vi "Calculate And Insert Biometry Parameter.vi"(8 "error in (no error)":errorcluster caption="错误输入（无错误）", 10 "Measure_No":i64, 11 "connection reference":T1) -> (0 "error out":errorcluster caption="错误输出")   [LabVIEW 2015, in "Boimetry Processing.lvlib"]
doc: "对当初测量第几次的所有测试信号进行计算。\n计算每次生物参数测量结果，测量结果错误判断。计算的结果添加到Biometry的Parameter数据库。\n输入：测量的第几次。"
uses:
  Boimetry Processing.lvlib
  <vilib>/addons/database/Connection.llb/Conn ObjectReference.ctl
  Database Processing/Support/Table/Biometry Parameter.ctl
  Utility VIs/Utility VIs.lvlib
  Digital Signal Processing/Digital Signal Processing.lvlib
  Database Processing/Database Processing.lvlib
  <vilib>/addons/database/NI_Database_API.lvlib
  Digital Image Processing/Digital Image Processing.lvlib
panel:
  # "Busy"
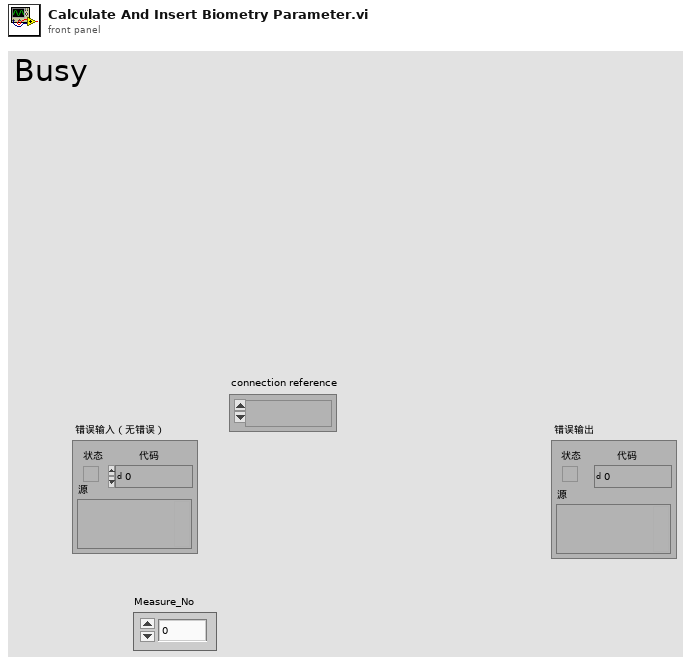
[diagram p1: front panel]
types:
  T1 = typedef "NI_Database_API.lvlib/Conn ObjectReference.ctl" = refnum<k1>
  T2 = typedef "Database Processing.lvlib/Biometry Parameter.ctl" = cluster{"Measure_ID":i64, "Central_Corneal_Thickness":sgl, "Anterior_Chamber_Depth":sgl, "Len_Thickness":sgl, "Retinal_Thickness":sgl, "Axis_Length":sgl, "Pupil_Diameter":sgl, "PCX":sgl, "PCY":sgl, "White_To_White":sgl, "ICX":sgl, "ICY":sgl, "Keratometric_flat":sgl, "Keratometric_steep":sgl, "Keratometric_Axis(flat)":sgl, "Keratometric_Axis(steep)":sgl, "Keratometric_AST":sgl}
  T3 = typedef "Database Processing.lvlib/Biometry Attribute.ctl" = cluster{"Measure_ID":i64, "Measure_No":i64, "Ordinal":i64, "L_Or_R":string}
  T4 = typedef "Digital Signal Processing.lvlib/DSP Configuration.ctl" = cluster{"Sampling Frequency":dbl, "filter type":T5, "RF Filter Low Frequency":dbl, "RF Filter High Frequency":dbl, "RF Filter Taps":i32, "window":T6, "RF window parameter":dbl, "filter type 2":T5, "Demodulated Filter Low Frequency":dbl, "Demodulated Filter HighFrequency":dbl, "Demodulated Filter Order":i32, "SPAN":i32, "Logarithmic Base":dbl, "Noise path":string, "Work position parameter":i32[]}
  T5 = typedef "NI_AALBase.lvlib/Filter Passband Type.ctl" = enum32{"Lowpass", "Highpass", "Bandpass", "Bandstop"}
  T6 = typedef "NI_AALPro.lvlib/windowTd.ctl" = u32
  T7 = typedef "Boimetry Processing.lvlib/Biometry Configuration.ctl" = cluster{"Interference Width":i32, "Interference Threshold":dbl, "Cornea Len Division":i32, "Correction Data 1st Path":string, "1st_Start_Position":dbl, "Correction Data 2nd Path":string, "2nd_Start_Position":dbl, "Index Corneal":dbl, "Index Water":dbl, "Index Len":dbl, "Working Position":cluster{"FirstStart":i32, "FirstEnd":i32, "SecondStart":i32, "SecondEnd":i32}}
  T8 = typedef "Digital Signal Processing.lvlib/DSP Parameter.ctl" = cluster{"RF":cluster{"filter structure":enum32{"IIR 2nd Order", "IIR 4th Order"}, "Reverse Coefficients":dbl[], "Forward Coefficients":dbl[]}, "IIR Filter Cluster":cluster{"filter structure":enum32{"IIR 2nd Order", "IIR 4th Order"}, "Reverse Coefficients":dbl[], "Forward Coefficients":dbl[]}, "Noise Signal":dbl[], "SPAN":i32, "Logarithmic Base":dbl}
  T9 = cluster{"filter structure":enum32{"IIR 2nd Order", "IIR 4th Order"}, "Reverse Coefficients":dbl[], "Forward Coefficients":dbl[]}
  T10 = typedef "Database Processing.lvlib/Biometry Data Path.ctl" = cluster{"Measure_ID":i64, "Ascan_data_Original":string, "picture_pupil_Original":string, "picture_WTW_Original":string, "Ascan_data_Processing":string, "picture_pupil_Processing":string, "picture_WTW_Processing":string, "picture_Processing_K":string, "picture_Processing_ALL":string}
  T11 = cluster{"FirstStart":i32, "FirstEnd":i32, "SecondStart":i32, "SecondEnd":i32}
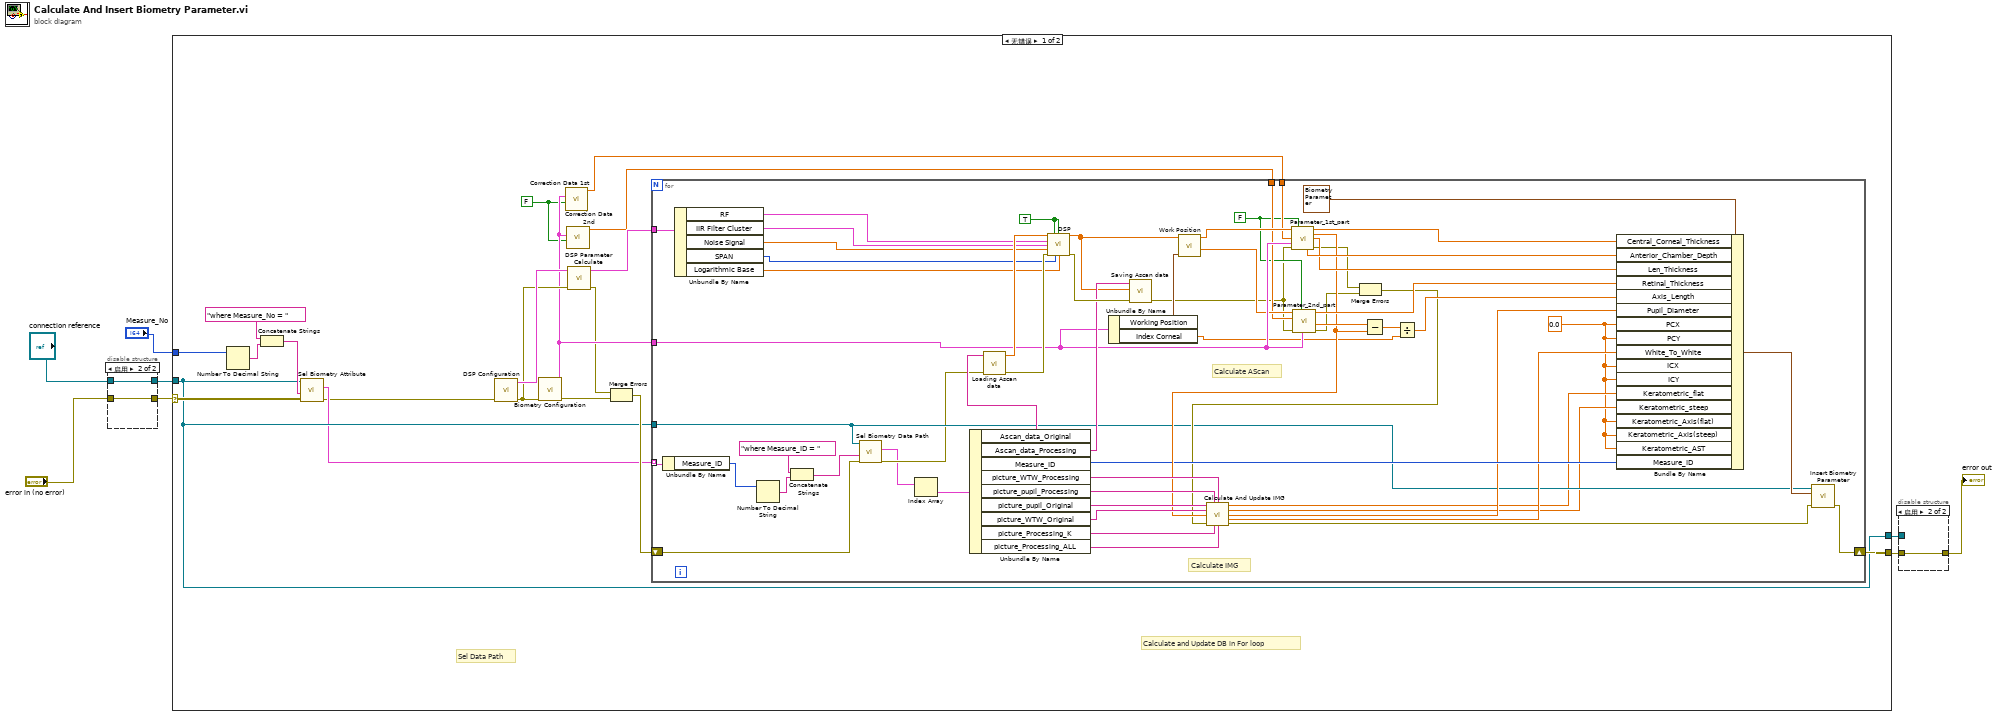
[diagram p0: block diagram]
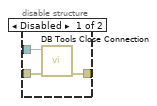
[diagram p2: hidden frame]
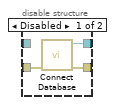
[diagram p3: hidden frame]
diagram:
  n1 = disable-structure shown="启用" {
    disable-tunnel: [w11 w13] -> w8
    disable-tunnel: "error in (no error)" -> [w10 w12]
    disable-tunnel: [w9 w12] -> w6
    disable-tunnel: "connection reference" -> [_ w13]
    frame Disabled {
      n2 = call "Connect Database.vi"("error in (no error)"=w10) -> ("error out"=w9:errorcluster, "connection reference"=w11:T1)  [unwired: 9 in]
    }
    frame Enabled {
    }
  }
  n3 = case shown="无错误" w6 {
    selector: w6 -> [w14 w92]
    tunnel: [w19 w92] -> w4
    tunnel: w8 -> [w16 w91]
    tunnel: [w16 w91] -> w3
    tunnel: "Measure_No" -> [w29 _]
    frame No Error {
      w22 = FALSE ("写入（非为读取）")
      # "Calculate and Update DB in For loop"
      # "Sel Data Path"
      n4 = Number To Decimal String(number=w29) -> (decimal integer string=w31:string)  [unwired: 1 in]
      n5 = Concatenate Strings("where Measure_No = " ("数据库配置.Condition"), w31) -> (w17:string)
      n6 = call "Sel Biometry Attribute.vi"("condition"=w17, "connection reference"=w16) -> ("Biometry Attribute"=w15:T3[])  [unwired: 8 in, 1 out]
      n7 = call "DSP Configuration.vi"("error in (no error)"=w14) -> ("error out"=w26:errorcluster, "DSP Parameter Output"=w28:T4)  [unwired: 9 in]
      n8 = call "Biometry Configuration.vi"("error in (no error)"=w26) -> ("error out"=w20:errorcluster, "Biometry Configuration"=w23:T7)  [unwired: 9 in]
      n9 = call "Correction Data 1st.vi"("写入（非为读取）"=w22, "Biometry Configuration"=w23) -> ("Output Correction Data"=w25:dbl[])  [unwired: 8 in, 1 out]
      n10 = call "Correction Data 2nd.vi"("写入（非为读取）"=w22, "Biometry Configuration"=w23) -> ("Output Correction Data"=w24:dbl[])  [unwired: 8 in, 1 out]
      n11 = call "DSP Parameter Calculate.vi"("error in (no error)"=w26, "DSP Configuration"=w28) -> ("error out"=w21:errorcluster, "DSP Parameter"=w27:T8)  [unwired: 8 in]
      n12 = Merge Errors(w21, w20) -> (w18:errorcluster)
      n13 = for {
        tunnel: w27 -> [w37]
        tunnel: w16 -> [w50]
        tunnel: w23 -> [w74]
        tunnel: w25 -> [w75]
        tunnel: w24 -> [w72]
        shift-right: [w51] -> w19
        shift-left: w18 -> [w49]
        tunnel: w15 -> [w45] mode=indexing
        w38 = sgl 0.0 ("PCX")
        w71 = FALSE
        w90 = TRUE
        # "Calculate IMG"
        # "Calculate AScan"
        n14 = Unbundle By Name(w45) -> ("Measure_ID"=w44:i64)
        n15 = Unbundle By Name(w37) -> ("RF"=w36:T9, "IIR Filter Cluster"=w35:T9, "Noise Signal"=w34:dbl[], "SPAN"=w33:i32, "Logarithmic Base"=w32:dbl)
        n16 = Number To Decimal String(number=w44) -> (decimal integer string=w47:string)  [unwired: 1 in]
        n17 = Concatenate Strings("where Measure_ID = " ("数据库配置.Condition"), w47) -> (w43:string)
        n18 = call "Sel Biometry Data Path.vi"("error in (no error)"=w49, "condition"=w43, "connection reference"=w50) -> ("error out"=w48:errorcluster, "Biometry Data Path"=w42:T10[])  [unwired: 7 in]
        n19 = Index Array(array=w42) -> (element=w41:T10)  [unwired: 1 in]
        n20 = Unbundle By Name(w41) -> ("Ascan_data_Original"=w82:string, "Ascan_data_Processing"=w81:string, "Measure_ID"=w60:i64, "picture_WTW_Processing"=w85:string, "picture_pupil_Processing"=w86:string, "picture_pupil_Original"=w88:string, "picture_WTW_Original"=w87:string, "picture_Processing_K"=w84:string, "picture_Processing_ALL"=w83:string)
        n21 = call "Loading Ascan data.vi"("error in (no error)"=w48, "名称或相对路径"=w82) -> ("error out"=w79:errorcluster, "first row"=w78:dbl[])  [unwired: 8 in]
        n22 = call "DSP.vi"("Input Signal"=w78, "Smooth(F : Don't)"=w90, "Minus Noise(F : Don't)"=w90, "RF"=w36, "IIR Filter Cluster"=w35, "Noise Signal"=w34, "error in (no error)"=w79, "SPAN"=w33, "Logarithmic Base"=w32) -> ("DSP signal"=w77:dbl[], "error out"=w89:errorcluster)  [unwired: 5 in]
        n23 = Unbundle By Name(w74) -> ("Working Position"=w80:T11, "Index Corneal"=w62:dbl)
        n24 = call "Saving Ascan data.vi"("error in (no error)"=w89, "Ascan Data"=w77, "名称或相对路径"=w81) -> ("error out"=w57:errorcluster)  [unwired: 8 in]
        n25 = call "Work Position.vi"("Working Position"=w80, "S"=w77) -> ("S_2nd_part"=w73:dbl[], "S_1st_part"=w76:dbl[])  [unwired: 4 in, 4 out]
        n26 = call "Parameter_1st_part.vi"("S"=w76, "测试"=w71, "Correction Data 1st"=w75, "Biometry Configuration"=w74, "Error In"=w57) -> ("角膜厚度"=w69:dbl, "开始位置"=w64:dbl, "晶体厚度"=w67:dbl, "前方深度"=w68:dbl, "Error Out"=w56:errorcluster)  [unwired: 4 in, 2 out]
        n27 = call "Parameter_2nd_part.vi"("Biometry Configuration"=w74, "测试？"=w71, "Error In"=w57, "Correction Data 2nd"=w72, "S"=w73) -> ("Error Out"=w55:errorcluster, "最值位置"=w65:dbl, "视网膜厚度"=w66:dbl)  [unwired: 3 in, 1 out]
        n28 = Merge Errors(w56, w55) -> (w54:errorcluster)
        n29 = call "Calculate And Update IMG.vi"("pictuer_pupil_Original"=w88, "pictuer_pupil_Processing"=w86, "pictuer_WTW_Processing"=w85, "pictuer_WTW_Original"=w87, "D"=w64, "error in (no error)"=w54, "picture_Processing_K"=w84, "picture_Processing_ALL"=w83) -> ("a"=w40:dbl, "b"=w39:dbl, "PD"=w59:dbl, "WTW"=w58:dbl, "error out"=w52:errorcluster)  [unwired: 3 in]
        n30 = Subtract(x=w65, y=w64) -> (x-y=w63:dbl)
        n31 = Divide(x=w63, y=w62) -> (x/y=w61:dbl)
        n32 = Bundle By Name(cluster=T2 {"Measure_ID"=0, "Central_Corneal_Thickness"=0.0, "Anterior_Chamber_Depth"=0.0, "Len_Thickness"=0.0, "Retinal_Thickness"=0.0, "Axis_Length"=0.0, "Pupil_Diameter"=0.0, "PCX"=0.0, "PCY"=0.0, "White_To_White"=0.0, "ICX"=0.0, "ICY"=0.0, "Keratometric_flat"=0.0, "Keratometric_steep"=0.0, "Keratometric_Axis(flat)"=0.0, "Keratometric_Axis(steep)"=0.0, "Keratometric_AST"=0.0} ("Biometry Parameter"), "Central_Corneal_Thickness"=w69, "Anterior_Chamber_Depth"=w68, "Len_Thickness"=w67, "Retinal_Thickness"=w66, "Axis_Length"=w61, "Pupil_Diameter"=w59, "PCX"=w38, "PCY"=w38, "White_To_White"=w58, "ICX"=w38, "ICY"=w38, "Keratometric_flat"=w40, "Keratometric_steep"=w39, "Keratometric_Axis(flat)"=w38, "Keratometric_Axis(steep)"=w38, "Keratometric_AST"=w38, "Measure_ID"=w60) -> (w53:T2)
        n33 = call "Insert Biometry Parameter.vi"("error in (no error)"=w52, "Biometry Parameter Input"=w53, "connection reference"=w50) -> ("error out"=w51:errorcluster)  [unwired: 8 in]
      }
    }
    frame Error {
    }
  }
  n34 = disable-structure shown="启用" {
    disable-tunnel: w4 -> [w95 w96]
    disable-tunnel: [w94 w96] -> w2
    disable-tunnel: w3 -> [w93 _]
    frame Disabled {
      n35 = call <vilib>:"DB Tools Close Connection.vi"("error in (no error)"=w95, "connection reference"=w93) -> ("error out"=w94:errorcluster)  [unwired: 5 in]
    }
    frame Enabled {
    }
  }
  "error out" <- w2
